vi "Search and add observer.vi"(8 "error in (no error)":errorcluster, 10 "Message in":refnum<class "InformMessage.lvclass">, 11 "Chat in":refnum<class "Chat.lvclass">) -> (0 "error out":errorcluster, 3 "Chat out":refnum<class "Chat.lvclass">)   [LabVIEW 2012, in "Chat.lvclass"]
uses:
  Chat.lvclass
  <vilib>/Distrio/Murmex/InformMessage/InformMessage.lvclass
  Chat.lvclass/Chat.ctl
  observers_cluster.ctl
  <vilib>/Distrio/Murmex/Message/Message.lvclass
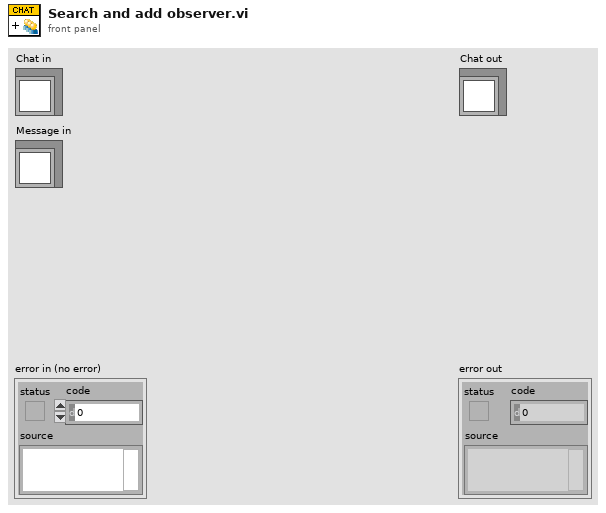
[diagram p1: front panel]
types:
  T1 = typedef "Chat.lvclass/observers_cluster.ctl" = cluster{"id":string, "writing":bool}
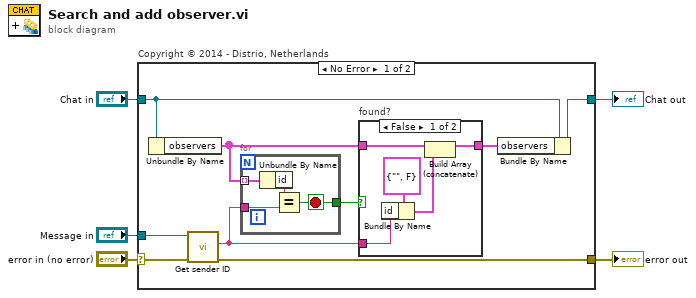
[diagram p0: block diagram]
diagram:
  n1 = case "Copyright © 2014 - Distrio, Netherlands" shown="No Error" "error in (no error)" {
    selector: "error in (no error)" -> [w14 w26]
    tunnel: [w13 w26] -> w4
    tunnel: [w7 w25] -> w2
    tunnel: "Chat in" -> [w8 w25]
    tunnel: "Message in" -> [w6 _]
    frame No Error {
      n2 = Unbundle By Name(w8) -> ("observers"=w11:T1[])
      n3 = call <vilib>:"Get sender ID.vi"("error in (no error)"=w14, "Message in"=w6) -> ("error out"=w13:errorcluster, "sender"=w10:string)  [unwired: 7 in, 1 out]
      n4 = for {
        tunnel: w11 -> [w24] mode=indexing
        tunnel: w10 -> [w22]
        tunnel: [w21] -> w12
        stop <- w21 stop-if-true
        n5 = Unbundle By Name(w24) -> ("id"=w23:string)
        n6 = Equal?(x=w23, y=w22) -> (x = y?=w21:bool)
      }
      n7 = case "found?" shown="False" w12 {
        tunnel: w11 -> [w19 w20]
        tunnel: w10 -> [w17 _]
        tunnel: [w15 w20] -> w9
        frame False {
          n8 = Bundle By Name(cluster=T1 {"id"="", "writing"=FALSE} ("observers"), "id"=w17) -> (w16:T1)
          n9 = Build Array (concatenate)(w19, w16) -> (w15:T1[])
        }
        frame True {
        }
      }
      n10 = Bundle By Name(cluster=w8, "observers"=w9) -> (w7:refnum<class "Chat.lvclass">)
    }
    frame Error {
    }
  }
  "error out" <- w4
  "Chat out" <- w2
